vi "OAT Timebase Plot (Filtered).vi"(0 "magnitudes":T4(array[cluster]) {"magnitude" format="%.2f"; "time/rev/rpm" format="%.2f"}, 2 "reset? (F)":bool, 3 "order to display":dbl=1.0 format="%.2f", 5 "phases [phase lag]":cluster{"time/rev/rpm":dbl[], "phase":dbl[]}[](array[cluster]) {"phase" format="%.2f"; "time/rev/rpm" format="%.2f"}, 7 "magnitude/phase position info":T1, 9 "revolutions to display [rev]":cluster{"start":dbl, "duration":dbl}={"start"=0.0, "duration"=8.0} {"duration" format="%.2f"; "start" format="%.2f"}, 11 "error in (no error)":errorcluster, 13 "view info":T3={"dB on? (F)"=FALSE, "unwrap phase? (T)"=TRUE, "unit in degree? (T)"=TRUE}, 14 "samples/rev wanted":i32=64) -> (4 "x-axis":T2, 6 "y-axis":T2, 15 "error out":errorcluster)   [LabVIEW 2017]
doc: "Draws a timebase plot with unfiltered or filtered data on an XY graph. The unfiltered data comes from the <B>even-angle signals</B> input, the filtered data from the <B>magnitudes</B> and <B>phases [phase lag]</B> inputs. The timebase plot displays the amplitude of a signal as a function of time and marks the tachometer trigger point on the plot. The data type you wire to the <B>even-angle signals</B> input determines the polymorphic instance to use."
uses:
  <vilib>/addons/Sound and Vibration/Order Analysis/Backward Compatibility/SubVIs/oa_Timebase Plot Control.ctl
  <vilib>/addons/Sound and Vibration/Order Analysis/Misc/OAT Position Info.ctl
  <vilib>/addons/Sound and Vibration/Order Analysis/Resample Order Tracking/SoundVib_Resampling.lvlib
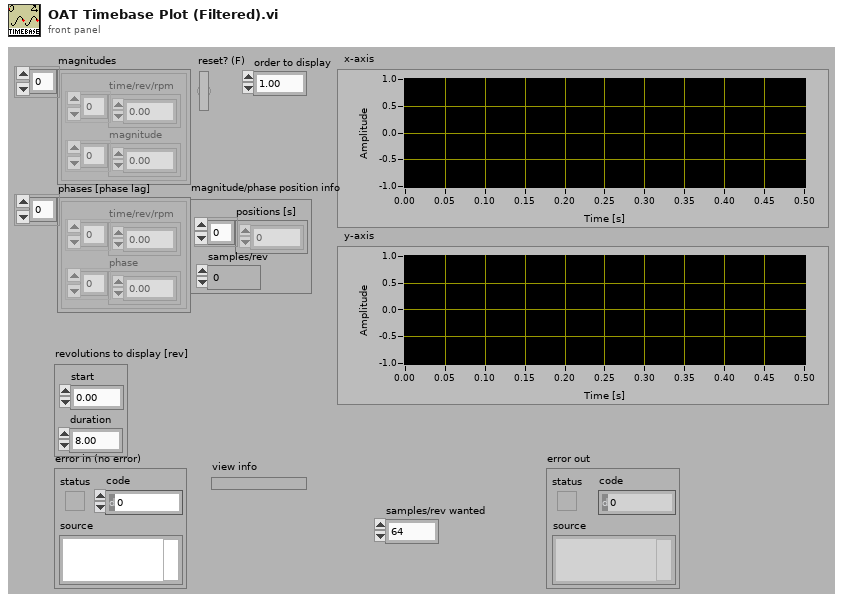
[diagram p1: front panel]
types:
  T1 = typedef "OAT Position Info.ctl" = cluster{"positions [s]":dbl[], "samples/rev":dbl}
  T2 = typedef "oa_Timebase Plot Control.ctl" = cluster{"X":dbl[], "Y":dbl[]}[]
  T3 = cluster{"dB on? (F)":bool, "unwrap phase? (T)":bool, "unit in degree? (T)":bool}
  T4 = cluster{"time/rev/rpm":dbl[], "magnitude":dbl[]}[]
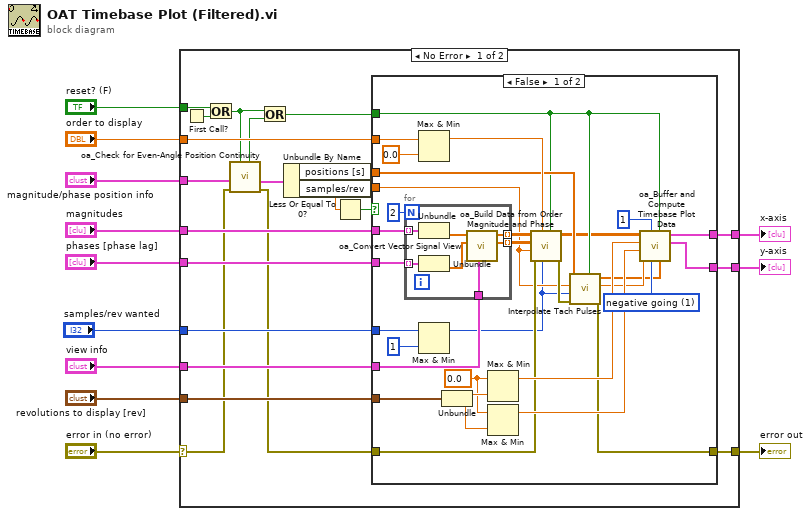
[diagram p0: block diagram]
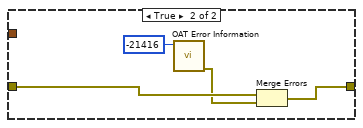
[diagram p2: hidden frame]
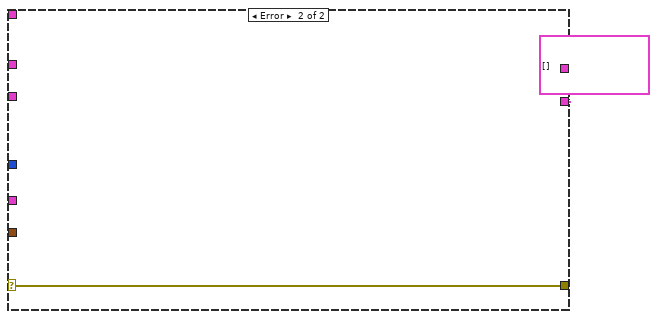
[diagram p3: hidden frame]
diagram:
  n1 = case shown="No Error" "error in (no error)" {
    selector: "error in (no error)" -> [w14 w77]
    tunnel: [w21 w77] -> w11
    tunnel: [w29 w76] -> w5
    tunnel: [w28 w76] -> w6
    tunnel: "magnitudes" -> [w33 _]
    tunnel: "phases [phase lag]" -> [w32 _]
    tunnel: "order to display" -> [w31 _]
    tunnel: "samples/rev wanted" -> [w30 _]
    tunnel: "revolutions to display [rev]" -> [w27 _]
    tunnel: "view info" -> [w26 _]
    tunnel: "magnitude/phase position info" -> [w19 _]
    tunnel: "reset? (F)" -> [w24 _]
    frame No Error {
      n2 = First Call?() -> (First Call?: T/F=w23:bool)
      n3 = Or(x=w24, y=w23) -> (x .or. y?=w17:bool)
      n4 = call <vilib>:"oa_Check for Even-Angle Position Continuity.vi"("reset in"=w17, "error in (no error)"=w14, "even-angle position info"=w19) -> ("error out"=w13:errorcluster, "even-angle position info dup"=w18:T1, "position not continuous"=w16:bool)  [unwired: 6 in]
      n5 = Or(x=w17, y=w16) -> (x .or. y?=w15:bool)
      n6 = Unbundle By Name(w18) -> ("positions [s]"=w20:dbl[], "samples/rev"=w22:dbl)
      n7 = Less Or Equal To 0?(x=w22) -> (x <= 0?=w25:bool)
      n8 = case shown="False" w25 {
        tunnel: w33 -> [w63 _]
        tunnel: w32 -> [w62 _]
        tunnel: w31 -> [w61 _]
        tunnel: w30 -> [w54 _]
        tunnel: [w52 _] -> w29
        tunnel: [w51 _] -> w28
        tunnel: w27 -> [w50 _]
        tunnel: w26 -> [w49 _]
        tunnel: w13 -> [w43 w74]
        tunnel: w15 -> [w36 _]
        tunnel: w22 -> [w41 _]
        tunnel: [w39 w72] -> w21
        tunnel: w20 -> [w38 _]
        frame False {
          w47 = u16 1 items=["positive going", "negative going"] ("trigger pulse direction")
          w55 = 0.0 ("y")
          n9 = for {
            N: 2 -> [_]
            tunnel: w63 -> [w71] mode=indexing
            tunnel: w62 -> [w70] mode=indexing
            tunnel: w49 -> [w67]
            tunnel: [w66] -> w46 mode=indexing
            tunnel: [w65] -> w45 mode=indexing
            n10 = Unbundle(w71) -> ("magnitude"=w69:dbl[])  [unwired: 1 out]
            n11 = Unbundle(w70) -> ("phase"=w68:dbl[])  [unwired: 1 out]
            n12 = call <vilib>:"oa_Convert Vector Signal View.vi"("view"=w67, "phase"=w68, "magnitude"=w69) -> ("phase out"=w65:dbl[], "magnitude out"=w66:dbl[])  [unwired: 7 in]
          }
          n13 = Max & Min(x=w61, y=0.0 ("t")) -> (max(x,y)=w44:dbl)  [unwired: 1 out]
          n14 = Max & Min(x=w54, y=1 ("x")) -> (max(x,y)=w40:i32)  [unwired: 1 out]
          n15 = Unbundle(w50) -> ("start"=w56:dbl, "duration"=w57:dbl)
          n16 = Max & Min(x=w55, y=w56) -> (max(x,y)=w59:dbl)  [unwired: 1 out]
          n17 = Max & Min(x=w55, y=w57) -> (max(x,y)=w58:dbl)  [unwired: 1 out]
          n18 = call <vilib>:"oa_Build Data from Order Magnitude and Phase.vi"("reset? (F)"=w36, "samples/revolution wanted"=w40, "order"=w44, "error in (no error)"=w43, "samples/revolution"=w41, "phase lag"=w45, "magnitude"=w46) -> ("error out"=w42:errorcluster, "order waveform"=w34:dbl[][])  [unwired: 2 in, 1 out]
          n19 = call <vilib>:"Interpolate Tach Pulses.vi"("reset? (True)"=w36, "error in (no error)"=w42, "pulse/revolution wanted"=w40, "pulse/revolution (1)"=w41, "pulse positions [s]"=w38) -> ("error out"=w39:errorcluster, "new pulse/revolution"=w37:dbl, "interpolated pulse positions[s]"=w35:dbl[])  [unwired: 4 in]
          n20 = call <vilib>:"oa_Buffer and Compute Timebase Plot Data.vi"("interpolated pulse positions[s]"=w35, "reset? (F)"=w36, "trigger pulse direction"=w47, "tach duty"=1, "actual samples/rev"=w37, "revolutions"=w58, "start"=w59, "order waveform"=w34) -> ("Y axis out"=w51:cluster{dbl[], dbl[]}[], "X axis out"=w52:cluster{dbl[], dbl[]}[])  [unwired: 2 in]
        }
        frame True {
          n21 = call <vilib>:"OAT Error Information.vi"("error code"=-21416) -> ("error out"=w73:errorcluster)  [unwired: 6 in]
          n22 = Merge Errors(w74, w73) -> (w72:errorcluster)
        }
      }
    }
    frame Error {
      w76 = cluster{"X":dbl[], "Y":dbl[]}[] [] ("X axis Plot")
    }
  }
  "error out" <- w11
  "y-axis" <- w6
  "x-axis" <- w5
